vi "Close.vi"(8 "error in (no error)":errorcluster, 11 "CS++Actor in":refnum<class "CS++Actor.lvclass">) -> (0 "error out":errorcluster, 3 "CS++Actor out":refnum<class "CS++Actor.lvclass">)   [LabVIEW 2014, in "CS++Actor.lvlib" / "CS++Actor.lvclass"]
doc: "Removes the References to this Actor."
uses:
  CS++Actor.lvclass
  CS++Actor.lvclass/CS++Actor.ctl
  CSPP_Method/CS++Method.lvclass
  CSPP_Message/CS++Message.lvclass
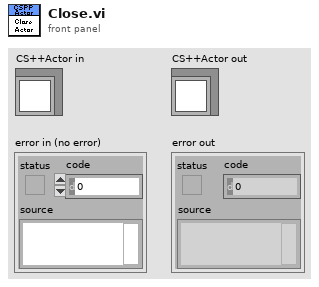
[diagram p1: front panel]
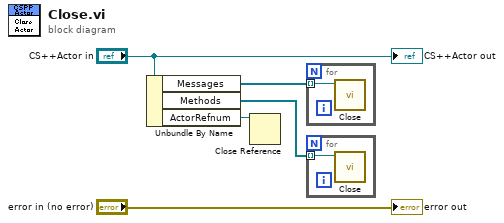
[diagram p0: block diagram]
diagram:
  n1 = Unbundle By Name("CS++Actor in") -> ("Messages"=w3:refnum<class "CS++Message.lvclass">[], "Methods"=w2:refnum<class "CS++Method.lvclass">[], "ActorRefnum"=w1:refnum<vi>)
  n2 = Close Reference(reference=w1) -> ()  [unwired: 1 in, 1 out]
  n3 = for {
    tunnel: w3 -> [w6] mode=indexing
    n4 = call-dynamic "Close.vi"("CS++Message in"=w6) -> ()  [unwired: 9 in, 2 out]
  }
  n5 = for {
    tunnel: w2 -> [w7] mode=indexing
    n6 = call-dynamic "Close.vi"("CS++Method in"=w7) -> ()  [unwired: 9 in, 2 out]
  }
  "error out" <- "error in (no error)"
  "CS++Actor out" <- "CS++Actor in"
